vi "Set Build Specification Version.vi"   [LabVIEW 2020, in "NI_App_Builder_API.lvlib"]
doc: "Sets the version information of a build specification. This VI sets the <B>Major, Minor, Fix</B>, and <B>Build</B> version numbers, which correspond to the version numbers on the <B>Version Information</B> page of the properties dialog box for the build specification. LabVIEW saves version information automatically only if you wire a path to this VI. Therefore, if you wire a project reference to this VI, you must manually save the project after you set the version information."
uses:
  <vilib>/AppBuilder/AB_API_Simple/NI_App_Builder_API.lvlib
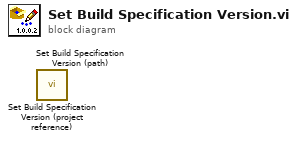
[diagram p0: block diagram]
diagram:
  n1 = call <vilib>:"Set Build Specification Version (project reference).vi"() -> ()  [unwired: 10 in, 2 out]
  n2 = call <vilib>:"Set Build Specification Version (path).vi"() -> ()  [unwired: 11 in, 1 out]
